vi "CRM-Config (TDT).vi"(8 "error in (no error)":errorcluster, 9 "TDT":T1, 10 "Num AI pts":i32, 11 "Sampling Rate (Hz)":dbl=20000.0) -> (0 "error out":errorcluster, 1 "Magnitude array":dbl[](array[numeric]), 3 "Freq resol (Hz)":dbl)   [LabVIEW 2020]
uses:
  epl-vi-lib/PXI DAQ VIs/TDT VIs/Typedefs/TDT-Device Config.ctl
  epl-vi-lib/PXI DAQ VIs/TDT VIs/Typedefs/TDT-Output source.ctl
  epl-vi-lib/PXI DAQ VIs/TDT VIs/Typedefs/TDT-Device ID.ctl
  epl-vi-lib/PXI DAQ VIs/TDT VIs/Typedefs/TDT-Input source.ctl
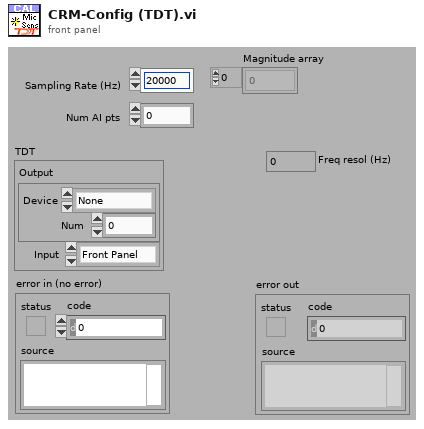
[diagram p1: front panel]
types:
  T1 = typedef "TDT-Device Config.ctl" = cluster{"Output":T2, "Input":T4}
  T2 = typedef "TDT-Output source.ctl" = cluster{"Device":T3, "Num":i32}
  T3 = typedef "TDT-Device ID.ctl" = enum16{"None", "PA5", "RP2", "RL2", "RA16", "RV8", "RX5", "RX6", "RX7", "RX8", "RZ2", "RZ5", "RZ6"}
  T4 = typedef "TDT-Input source.ctl" = enum16{"Front Panel", "RA4LI", "RA16LI"}
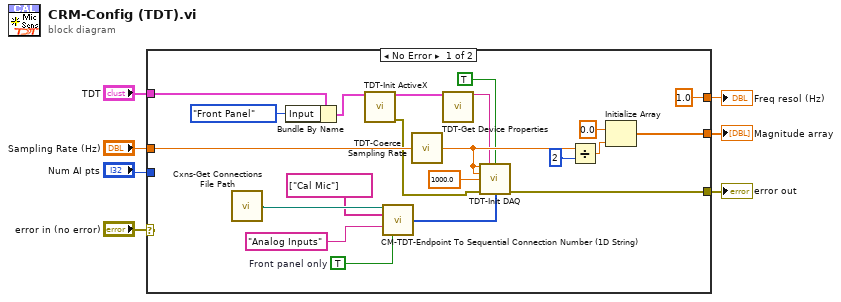
[diagram p0: block diagram]
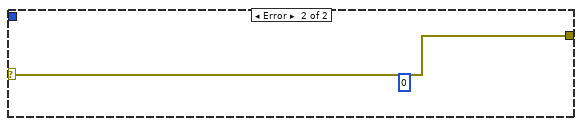
[diagram p2: hidden frame]
diagram:
  n1 = case shown="No Error" "error in (no error)" {
    selector: "error in (no error)" -> [_ w29]
    tunnel: [w25 w29] -> w6
    tunnel: "Num AI pts" -> [_ _]
    tunnel: "Sampling Rate (Hz)" -> [w24 _]
    tunnel: [1.0 _] -> w3
    tunnel: [w26 _] -> w2
    tunnel: "TDT" -> [w20 _]
    frame No Error {
      w13 = TRUE  # Front panel only
      n2 = call "Cxns-Get Connections File Path.vi"() -> ("Path Out"=w17:path)  [unwired: 1 in]
      n3 = Bundle By Name(cluster=w20, "Input"=enum16{"Front Panel", "RA4LI", "RA16LI"}."Front Panel") -> (w10:T1)
      n4 = call "TDT-Init ActiveX.vi"("TDT-Device Config"=w10) -> ("TDT-Device Config out"=w9:T1, "error out"=w8:errorcluster)  [unwired: 11 in, 2 out]
      n5 = call "CM-TDT-Endpoint To Sequential Connection Number (1D String).vi"("Path In"=w17, "Endpoints"=string[] ["Cal Mic"], "Section"="Analog Inputs", "Front panel only"=w13) -> ("SeqCxnNum"=w12:i32[])  [unwired: 9 in, 2 out]
      n6 = call "TDT-Coerce Sampling Rate.vi"("Fs (Hz)"=w24) -> ("Coerced"=w21:dbl)
      n7 = call "TDT-Get Device Properties.vi"("TDT-Device Config"=w9) -> ("Circuit File"=w19:string)  [unwired: 9 in, 5 out]
      n8 = call "TDT-Init DAQ.vi"("AO Fs (Hz)"=w21, "Circuit"=w19, "AI only"=TRUE, "AI Fs (Hz)"=w21, "T (ms)"=1000.0, "error in (no error)"=w8, "AI Channels"=w12) -> ("error out"=w25:errorcluster)  [unwired: 4 in, 4 out]
      n9 = Divide(x=w21, y=2) -> (x/y=w11:dbl)
      n10 = Initialize Array(0.0 ("element"), w11) -> (w26:dbl[])
    }
    frame Error {
      (unwired) 0
    }
  }
  "error out" <- w6
  "Freq resol (Hz)" <- w3
  "Magnitude array" <- w2
